vi "LaserCal-Compute I-O.vi"(9 "I-O Data in":T1, 11 "error in (no error)":errorcluster, 12 "Time Graph":refnum<vi>, 13 "I-O":refnum<vi>) -> (10 "I-O Data out":T1, 15 "error out":errorcluster)   [LabVIEW 2015]
uses:
  Typedefs/LaserCal-Data (I-O).ctl
  <vilib>/Analysis/baseanly.llb/Mean (DBL).vi
  Utility VIs/Array Manipulation VIs/Irregular Array Subset (DBL).vi
  <vilib>/Analysis/NI_AALBase.lvlib
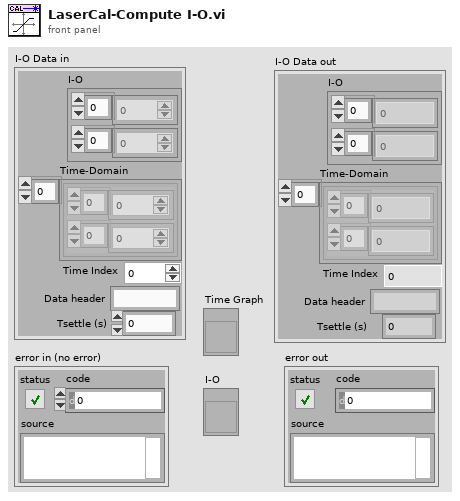
[diagram p1: front panel]
types:
  T1 = typedef "LaserCal-Data (I-O).ctl" = cluster{"I-O":cluster{dbl[], dbl[]}, "Time-Domain":cluster{dbl[], dbl[]}[], "Time Index":i32, "Data header":string, "Tsettle (s)":dbl}
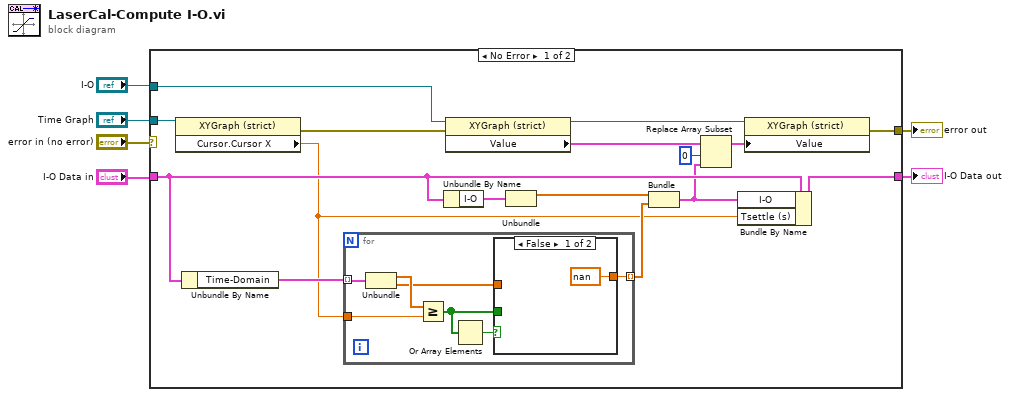
[diagram p0: block diagram]
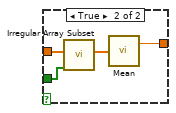
[diagram p2: hidden frame]
diagram:
  n1 = case shown="No Error" "error in (no error)" {
    selector: "error in (no error)" -> [_ w36]
    tunnel: [w15 w36] -> w3
    tunnel: "Time Graph" -> [w21 _]
    tunnel: "I-O" -> [w13 _]
    tunnel: "I-O Data in" -> [w20 w35]
    tunnel: [w16 w35] -> w1
    frame No Error {
      n2 = property class="XYGraph (strict)"(reference=w21) -> (error out=w14:errorcluster, "Cursor.Cursor X"=w7:dbl)  [unwired: 1 in, 1 out]
      n3 = Unbundle By Name(w20) -> ("Time-Domain"=w22:cluster{dbl[], dbl[]}[])
      n4 = for {
        tunnel: w22 -> [w29] mode=indexing
        tunnel: w7 -> [w27]
        tunnel: [w23] -> w17 mode=indexing
        n5 = Unbundle(w29) -> (w28:dbl[], w25:dbl[])
        n6 = Greater Or Equal?(x=w28, y=w27) -> (x >= y?=w26:bool[])
        n7 = Or Array Elements(Boolean array=w26) -> (logical OR=w24:bool)
        n8 = case shown="False" w24 {
          tunnel: w26 -> [_ w34]
          tunnel: w25 -> [_ w33]
          tunnel: [nan ("mean") w31] -> w23
          frame False {
          }
          frame True {
            n9 = call-poly "Irregular Array Subset.vi"("Mask"=w34, "Array"=w33) -> ("Array Subset"=w32:dbl[])  [unwired: 8 in, 1 out]
            n10 = call-poly <vilib>:"Mean.vi"("X"=w32) -> ("mean"=w31:dbl)  [unwired: 1 out]
          }
        }
      }
      n11 = Unbundle By Name(w20) -> ("I-O"=w19:cluster{dbl[], dbl[]})
      n12 = property class="XYGraph (strict)"(reference=w13, error in=w14) -> (reference out=w12:refnum<vi>, "Value"=w10:cluster{"Frequency":dbl[], "Frequency":dbl[]}[])  [unwired: 1 out]
      n13 = Unbundle(w19) -> (w18:dbl[])  [unwired: 1 out]
      n14 = Bundle(w18, w17) -> (w11:cluster{dbl[], dbl[]})  [unwired: 1 in]
      n15 = Replace Array Subset(array=w10, new element=w11, index=0) -> (w9:cluster{"Frequency":dbl[], "Frequency":dbl[]}[])
      n16 = Bundle By Name(cluster=w20, "I-O"=w11, "Tsettle (s)"=w7) -> (w16:T1)
      n17 = property class="XYGraph (strict)"(reference=w12, "Value"=w9) -> (error out=w15:errorcluster)  [unwired: 1 in, 1 out]
    }
    frame Error {
    }
  }
  "error out" <- w3
  "I-O Data out" <- w1
